vi "Periodic Tasks.vi"(8 "error in":errorcluster) -> ()   [LabVIEW 2017]
doc: "This VI runs in parallel to other tasks. It can contain as many user-defined periodic loops as you need. These can carry out PID or other sorts of timed response."
uses:
  SwerveLibrary/Sensors.ctl
  SwerveLibrary/Drive Motors.ctl
  SwerveLibrary/Swerve Motors.ctl
  Public/Documents/Cross The Road Electronics/Phoenix-LabVIEW/Pigeon IMU/CTRE_PigeonIMU_GetYPR.vi
  Public/Documents/Cross The Road Electronics/Phoenix-LabVIEW/Motor Controller/Get/CTRE_Phoenix_MotorController_GetSelectedSensorData.vi
  Robot Global Data.vi
  SwerveLibrary/Huskie Swerve.lvlib
panel:
  out "all currents (A)":dbl[](array[numeric])
  out "Yaw Pitch Roll":cluster{"Yaw":dbl, "Pitch":dbl, "Roll":dbl}
  out "Swerve Positions":i32[](array[numeric])
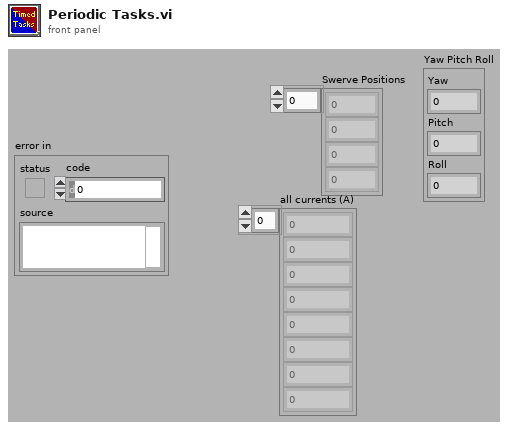
[diagram p1: front panel]
types:
  T1 = typedef "Huskie Swerve.lvlib/Sensors.ctl" = enum16{"Gyro", "Vision USB", "Button Pressed", "Other sensor", "Generic Sensor"}
  T2 = typedef "Huskie Swerve.lvlib/Swerve Motors.ctl" = enum16{"Swerve 1", "Swerve 2", "Swerve 3", "Swerve 4"}
  T3 = typedef "WPI_MotorControlDeviceRef.ctl" = cluster{"DeviceStatus":errorcluster, "Type":T4, "PWM":cluster{"PWM Channel":T5, "DeadBand":T6}, "CAN":cluster{"Device Number":u8, "SetOutput VI Ref":variant, "GetOutput VI Ref":variant, "Enable VI Ref":variant, "Disable VI Ref":variant, "Data":variant}, "Invert":bool, "DIO PWM":cluster{"PWM \"Enable\" Channel":T5, "DIOChannel":T7, "PWM Rate":dbl}}
  T4 = typedef "WPI_MotorControlType.ctl" = enum16{"PWM", "CAN", "DIO PWM"}
  T5 = typedef "FPGA_DIOPWMChannel.ctl" = enum8{"PWM 0", "PWM 1", "PWM 2", "PWM 3", "PWM 4", "PWM 5", "PWM 6", "PWM 7", "PWM 8", "PWM 9", "PWM MXP 0", "PWM MXP 1", "PWM MXP 2", "PWM MXP 3", "PWM MXP 4", "PWM MXP 5", "PWM MXP 6", "PWM MXP 7", "PWM MXP 8", "PWM MXP 9", "Invalid"}
  T6 = typedef "WPI_PWMDeadband.ctl" = cluster{"Name":string, "maxPositivePwm":i32, "minPositivePwm":i32, "centerPwm":i32, "maxNegativePwm":i32, "minNegativePwm":i32, "angularRange":u16}
  T7 = typedef "FPGA_DIOChannel.ctl" = enum8{"DIO 0", "DIO 1", "DIO 2", "DIO 3", "DIO 4", "DIO 5", "DIO 6", "DIO 7", "DIO 8", "DIO 9", "DIO MXP 0", "DIO MXP 1", "DIO MXP 2", "DIO MXP 3", "DIO MXP 4", "DIO MXP 5", "DIO MXP 6", "DIO MXP 7", "DIO MXP 8", "DIO MXP 9", "DIO MXP 10", "DIO MXP 11", "DIO MXP 12", "DIO MXP 13", "DIO MXP 14", "DIO MXP 15", "SPI Port CS1", "SPI Port CS2", "SPI Port CS3", "SPI Port MISO", "SPI Port MOSI", "Invalid"}
  T8 = typedef "Huskie Swerve.lvlib/Drive Motors.ctl" = enum16{"Drive 1", "Drive 2", "Drive 3", "Drive 4"}
  T9 = typedef "CTRE_PigeonIMU_DeviceRef.ctl" = cluster{"DeviceStatus":errorcluster, "Device Number":u8, "Type":T10, "Device ID":u32, "Handle":u64, "UsageFrame":u32, "Library Path":path}
  T10 = typedef "CTRE_PigeonIMU_ConnectionType.ctl" = u32
  T11 = cluster{"X":dbl, "Y":dbl, "Z":dbl, "X Drive":bool, "Field Relative":bool, "Actuate Grabber":bool, "Inverse Drive":bool}
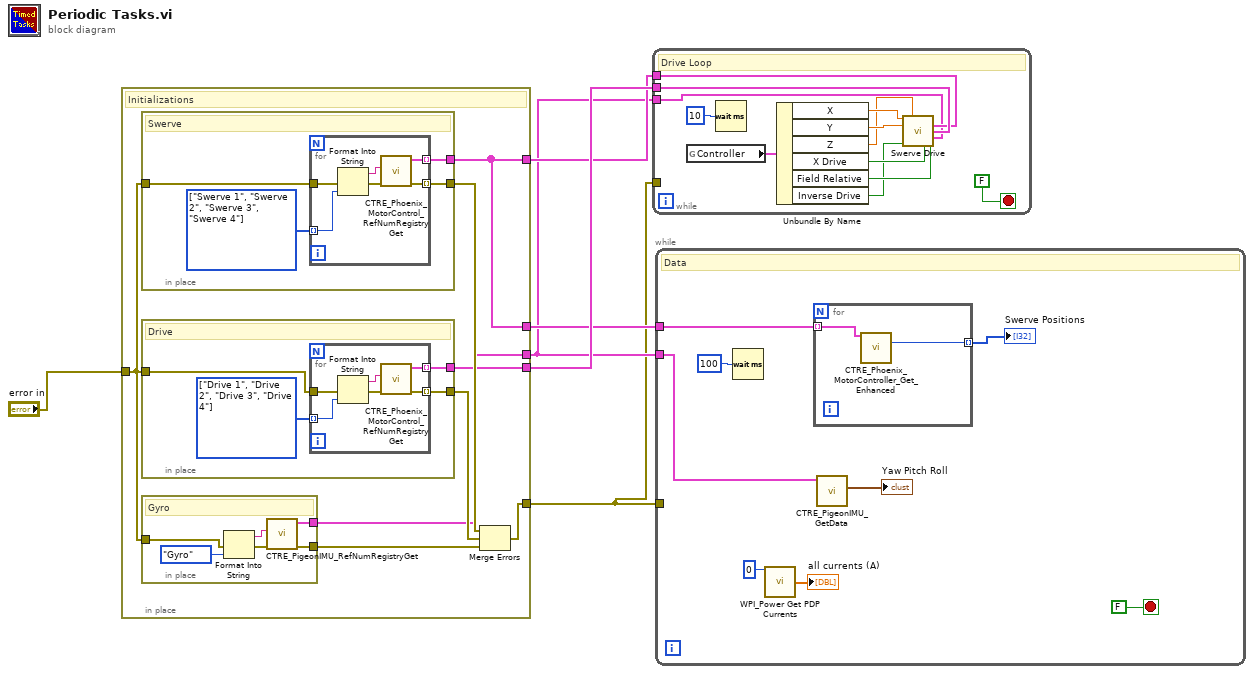
[diagram p0: block diagram]
diagram:
  n1 = in-place {
    in-place-border: "error in" -> [w11]
    in-place-border: [w10] -> w5
    in-place-border: [w8] -> w4
    in-place-border: [w9] -> w2
    in-place-border: [w8] -> w3
    in-place-border: [w7] -> w1
    # "Initializations"
    n2 = in-place {
      in-place-border: [w33] -> w14
      in-place-border: w11 -> [w32]
      in-place-border: [w31] -> w8
      w34 = T2[] [enum."Swerve 1", enum."Swerve 2", enum."Swerve 3", enum."Swerve 4"] items=["Swerve 1", "Swerve 2", "Swerve 3", "Swerve 4"] ("Array")
      # "Swerve"
      n3 = for {
        tunnel: w34 -> [w39] mode=indexing
        tunnel: [w38] -> w33 mode=indexing
        tunnel: w32 -> [w37]
        tunnel: [w35] -> w31 mode=indexing
        n4 = Format Into String(error in=w37, w39) -> (resulting string=w40:string, error out=w36:errorcluster)  [unwired: 2 in]
        n5 = call "CTRE_Phoenix_MotorControl_RefNumRegistryGet.vi"("error in (no error)"=w36, "refnum name"=w40) -> ("error out"=w38:errorcluster, "PhoenixMotorControlDevRef"=w35:T3)  [unwired: 8 in]
      }
    }
    n6 = in-place {
      in-place-border: [w23] -> w13
      in-place-border: w11 -> [w22]
      in-place-border: [w21] -> w10
      w24 = T8[] [enum."Drive 1", enum."Drive 2", enum."Drive 3", enum."Drive 4"] items=["Drive 1", "Drive 2", "Drive 3", "Drive 4"] ("Array")
      # "Drive"
      n7 = for {
        tunnel: w24 -> [w29] mode=indexing
        tunnel: [w28] -> w23 mode=indexing
        tunnel: w22 -> [w27]
        tunnel: [w25] -> w21 mode=indexing
        n8 = Format Into String(error in=w27, w29) -> (resulting string=w30:string, error out=w26:errorcluster)  [unwired: 2 in]
        n9 = call "CTRE_Phoenix_MotorControl_RefNumRegistryGet.vi"("error in (no error)"=w26, "refnum name"=w30) -> ("error out"=w28:errorcluster, "PhoenixMotorControlDevRef"=w25:T3)  [unwired: 8 in]
      }
    }
    n10 = in-place {
      in-place-border: [w17] -> w12
      in-place-border: w11 -> [w16]
      in-place-border: [w15] -> w9
      # "Gyro"
      n11 = Format Into String(error in=w16, Sensors."Gyro" ("Enum")) -> (resulting string=w18:string, error out=w20:errorcluster)  [unwired: 2 in]
      n12 = call "CTRE_PigeonIMU_RefNumRegistryGet.vi"("error in (no error)"=w20, "refnum name"=w18) -> ("error out"=w17:errorcluster, "PigeonIMUDevRef"=w15:T9)  [unwired: 8 in]
    }
    n13 = Merge Errors(w14, w13, w12) -> (w7:errorcluster)
  }
  n14 = while {
    tunnel: w5 -> [w52]
    tunnel: w4 -> [w51]
    tunnel: w2 -> [w50]
    tunnel: w1 -> [_]
    stop <- FALSE stop-if-true
    # "Drive Loop"
    n15 = global read "Robot Global Data.vi" "Controller"() -> (w47:T11)
    n16 = Wait (ms)(milliseconds to wait=u32 10) -> ()  [unwired: 1 out]
    n17 = Unbundle By Name(w47) -> ("X"=w46:dbl, "Y"=w45:dbl, "Z"=w44:dbl, "X Drive"=w43:bool, "Field Relative"=w42:bool, "Inverse Drive"=w41:bool)
    n18 = call "Swerve Drive.vi"("X"=w46, "Z"=w44, "Y"=w45, "Swerve Dev Ref"=w51, "Drive Dev Ref"=w52, "PigeonIMUDevRef"=w50, "Reverse Drive"=w41, "X Drive"=w43, "Field Relative Active"=w42) -> ()  [unwired: 6 in, 1 out]
  }
  n19 = while {
    tunnel: w3 -> [w60]
    tunnel: w2 -> [w57]
    tunnel: w1 -> [_]
    stop <- FALSE stop-if-true
    # "Data"
    n20 = Wait (ms)(milliseconds to wait=u32 100) -> ()  [unwired: 1 out]
    n21 = call <vilib>:"WPI_Power Get PDP Currents.vi"("Power Distribution Panel (0)"=u8 0) -> ("all currents (A)"=→"all currents (A)":dbl[])  [unwired: 12 in, 2 out]
    n22 = for {
      tunnel: w60 -> [w62] mode=indexing
      tunnel: [w61] -> w59 mode=indexing
      n23 = call-poly <vilib>:"CTRE_Phoenix_MotorController_Get_Enhanced.vi"("PhoenixMotorControlDevRef"=w62) -> ("Position (Raw Sensor Units)"=w61:i32)  [unwired: 11 in, 3 out]
    }
    "Swerve Positions" <- w59
    n24 = call-poly "CTRE_PigeonIMU_GetData.vi"("PigeonIMUDevRef"=w57) -> ("Yaw Pitch Roll"=→"Yaw Pitch Roll":cluster{"Yaw":dbl, "Pitch":dbl, "Roll":dbl})  [unwired: 8 in, 2 out]
  }
